vi "_pickOutColsOfCheck_EEPROM_VNA_wmg.vi"(3 "sys_index":i32, 4 "indexToBeFind":i32, 5 "EEPROMCheck":string[][](array[string])=[["0", "1", "0", "3"], ["0", "1", "10", "14"], ["0", "3", "2", "4"], ["1", "1", "0", "3"], ["1", "1", "10", "14"], ["1", "3", "2", "4"]]) -> (0 "x != y?":bool, 1 "output":i32[][](array[numeric]), 2 "output":string[][](array[string]))   [LabVIEW 2011]
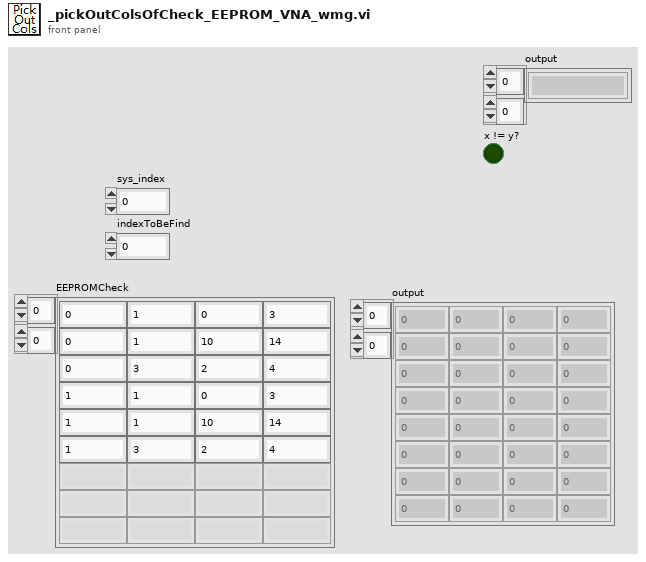
[diagram p1: front panel]
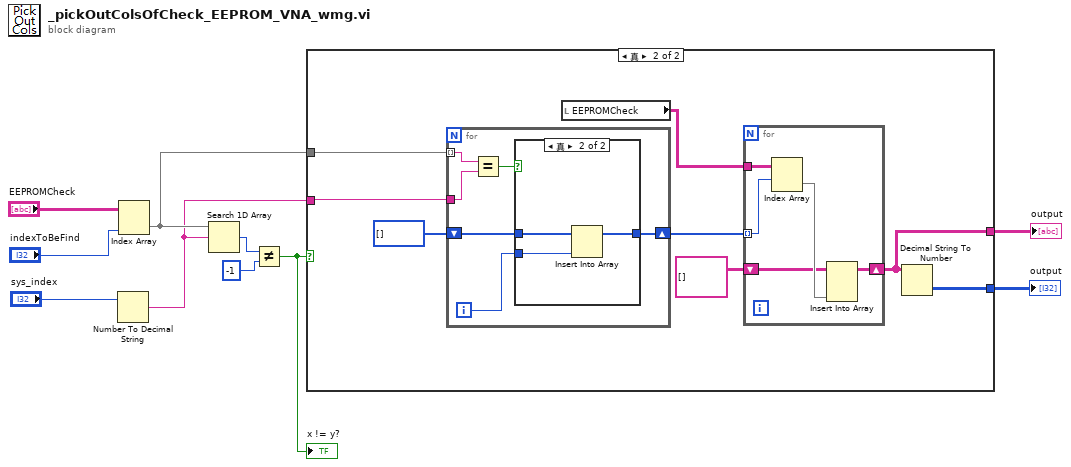
[diagram p0: block diagram]
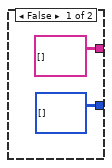
[diagram p2: hidden frame]
diagram:
  n1 = Number To Decimal String(number="sys_index") -> (decimal integer string=w3:string)  [unwired: 1 in]
  n2 = Index Array(array="EEPROMCheck", index (col)="indexToBeFind") -> (element=w4:string[])  [unwired: 1 in]
  n3 = Search 1D Array(1D array=w4, element=w3) -> (index of element=w7:i32)  [unwired: 1 in]
  n4 = Not Equal?(x=w7, y=-1) -> (x != y?=w5:bool)
  "x != y?" <- w5
  n5 = case shown="真" w5 {
    tunnel: w4 -> [_ w16]
    tunnel: w3 -> [_ w15]
    tunnel: [i32[][] [] w14] -> w2
    tunnel: [string[][] [] ("EEPROMCheck 2") w13] -> w1
    frame False {
    }
    frame True {
      n6 = for {
        tunnel: w16 -> [w31] mode=indexing
        tunnel: w15 -> [w30]
        shift-right: [w27] -> w19
        shift-left: i32[] [] -> [w28]
        i -> [w26]
        n7 = Equal?(x=w31, y=w30) -> (x = y?=w29:bool)
        n8 = case shown="真" w29 {
          tunnel: w28 -> [w32 w35]
          tunnel: [w32 w34] -> w27
          tunnel: w26 -> [_ w33]
          frame False {
          }
          frame True {
            n9 = Insert Into Array(array=w35, new element=w33) -> (w34:i32[])  [unwired: 1 in]
          }
        }
      }
      n10 = local read "EEPROMCheck"() -> (w18:string[][])
      n11 = for {
        tunnel: w19 -> [w24] mode=indexing
        tunnel: w18 -> [w25]
        shift-right: [w21] -> w13
        shift-left: string[][] [] ("EEPROMCheck 2") -> [w22]
        n12 = Index Array(array=w25, index (row)=w24) -> (element=w23:string[])  [unwired: 1 in]
        n13 = Insert Into Array(array=w22, new element=w23) -> (w21:string[][])  [unwired: 2 in]
      }
      n14 = Decimal String To Number(string=w13) -> (number=w14:i32[][])  [unwired: 2 in, 1 out]
    }
  }
  "output" <- w2
  "output" <- w1
